vi "mmWave TX driver (FPGA).vi"() -> ()   [LabVIEW 2019]
uses:
  SubVIs/Tone Generator/Channel Control.ctl
  SubVIs/Sync/Sync Control.ctl
  SubVIs/Sync/Sync Measurements.ctl
  <instrlib>/_niInstr/DSP/v1/Shared/Public/IQ Impairments.ctl
  <instrlib>/_niInstr/DSP/v1/Shared/Public/Filter Coefficients.ctl
  Host/SubVIs/Low-level/TypeDefs/Gain Setting.ctl
  <instrlib>/niMmWave/ni3620/Config/v1/FPGA/Public/Typedefs/TX1 RX1 Port.ctl
  SubVIs/Utility/FPGA driver trigger destination.ctl
  SubVIs/Utility/FPGA driver trigger source.ctl
  SubVIs/DRAM burst sequencer/DRAM mode.ctl
  SubVIs/DRAM burst sequencer/SegementSequencer_class/FPGA sequencer states.ctl
  SubVIs/DRAM burst sequencer/Burst memo.ctl
  SubVIs/DRAM burst sequencer/DRAM resources.ctl
  <instrlib>/_niInstr/Memory/v1/FPGA/DRAM U512/niInstr Memory DRAM U512 v1 FPGA.lvclass
  <instrlib>/_niInstr/Memory/v1/FPGA/BRAM U512/niInstr Memory BRAM U512 v1 FPGA.lvclass
  <vilib>/Platform/TimedLoop/XDataNode/timing_clust.ctl
  <vilib>/Platform/TimedLoop/XDataNode/nitl_modes.ctl
  <vilib>/Platform/TimedLoop/XDataNode/wakeup.ctl
  <instrlib>/_niInstr/DSP/v1/Shared/Public/IQ Data.ctl
  <instrlib>/_niInstr/Memory/v1/FPGA/DRAM U512/Public/Create.vi
  <instrlib>/_niInstr/Memory/v1/FPGA/BRAM U512/Public/Create.vi
  <vilib>/rvi/Emulation/niFpgaSctlEmulationGetInTimedLoop.vi
  <vilib>/rvi/Emulation/niFpgaEmulationReportErrorSimple.vi
  <vilib>/rvi/Emulation/niFpgaGetClockAttributes.vi
  <vilib>/rvi/Emulation/niFpgaCriticalErrorInLSC.vi
  <vilib>/rvi/Emulation/niFpgaProcessEmulError.vi
  <vilib>/rvi/eio/common/nirviEmuTemplateMethod_errors.vi
  SubVIs/Misc/Globals.vi
  <vilib>/rvi/DataTransferAndStorage/Container/Common/niFpgaContainerGetUniqueNameForEmu.vi
  <vilib>/rvi/DataTransferAndStorage/Container/Common/niFpgaContainerSetEmuInfo.vi
  <vilib>/rvi/eio/common/nirviEmuReportErrorAndStop.vi
  <vilib>/rvi/Emulation/niFpgaEmulationIsFPGAContextNoSignature.vi
  <vilib>/rvi/errors/niFpgaSetErrorForExecOnDevCompSimple.vi
  <vilib>/rvi/FIFO/Fifo_Resource/nirvififoEmulationSetSize.vi
  <vilib>/rvi/FIFO/Fifo_Resource/nirviFifoEmulationQueueMgr.vi
  <instcachedir>/0/nirviFifoEmulationQueueMgr_E5CAEC123FF24DC58D834DCA3CDAA9B5.lvgen/nirviFifoEmulationQueueMgr_E5CAEC123FF24DC58D834DCA3CDAA9B5_008.vi
  <vilib>/Utility/error.llb/Clear Errors.vi
  <vilib>/rvi/FIFO/Fifo_Resource/nirvififoEmulationCreateLock.vi
  <vilib>/rvi/FIFO/Fifo_Resource/nirvififoEmulationObtainLock.vi
  <vilib>/rvi/FIFO/Fifo_Resource/nirvififoEmulationReleaseLock.vi
  <vilib>/rvi/occurrence/nirviWaitOnOccurrenceBase.vi
  <vilib>/rvi/errors/nirviReportUnexpectedCaseInternalError.vi
  <vilib>/rvi/errors/nirviReportUnexpectedCaseInternalError (U32).vi
  <vilib>/rvi/FIFO/Fifo_Resource/nirvififoEmulationDetermineInputValidOut.vi
  <vilib>/rvi/DataTransferAndStorage/Container/Common/niFpgaContainerExecOnDevCompGetState.vi
  <instcachedir>/0/nirviFifoEmulationQueueMgr_E5CAEC123FF24DC58D834DCA3CDAA9B5.lvgen/nirviFifoEmulationQueueMgr_E5CAEC123FF24DC58D834DCA3CDAA9B5_011.vi
  <vilib>/rvi/interface/RandomDataEmulation/niFpgaRandomDataHandleErrors.vi
  <instrlib>/_niInstr/Basic Elements/v1/FPGA/Private/Count Up U64.vi
  <vilib>/Platform/TimedLoop/XDataNode/XDataNode.xnode
  <vilib>/eio/EIONode/EIONode.xnode
  <vilib>/rvi/LocalResourceManager/LocalResourceManager.xnode
  <vilib>/rvi/DataTransferAndStorage/Container/XNode/niFpgaContainer.xnode
  <vilib>/rvi/FIFO/Fifo_Resource/nirvififoEmulationRead.vi
  <vilib>/rvi/FIFO/Fifo_Resource/nirvififoEmulationWrite.vi
  <vilib>/eio/EIOMethodNode/EIOMethodNode.xnode
  <vilib>/rvi/FIFO/Fifo_Resource/niFpgaFifoEmulationRefIn.vi
  SubVIs/DRAM burst sequencer/SegementSequencer_class/SegmentSequencer.lvclass
  <vilib>/Platform/TimedLoop/XDataNode/XDNodeRunTimeDep.lvlib
  <instrlib>/_niInstr/Basic Elements/v1/FPGA/niInstr Basic Elements v1 FPGA.lvlib
  <instrlib>/_niInstr/Data Formatting/v1/FPGA/niInstr Data Formatting v1 FPGA.lvlib
  <vilib>/rvi/Memory/Memory_Emulation/nirvimemoryFastEmulation.vi
  <vilib>/rvi/Memory/Memory_Emulation/nirvimemoryEmulation.vi
  <instrlib>/_niInstr/Basic Elements/v1/FPGA/Private/Count Up U16.vi
  <instrlib>/_niInstr/DSP/v1/Shared/niInstr DSP v1 Shared.lvlib
  <instrlib>/niMmWave/ni3620/Config/v1/FPGA/niMmWave Config v1 FPGA.lvlib
  <vilib>/rvi/interface/RandomDataEmulation/nirviRandomDataFpgaMultiElementTemplate.vi
  SubVIs/Utility/FPGA Utility.lvlib
  <instrlib>/_niInstr/Memory/v1/FPGA/DRAM/niInstr Memory DRAM v1 FPGA.lvclass
  SubVIs/DRAM burst sequencer/TX burst sequencer.lvlib
  <instrlib>/_niInstr/Memory/v1/FPGA/BRAM/niInstr Memory BRAM v1 FPGA.lvclass
  <instrlib>/_niInstr/Data Formatting/v1/FPGA/Private/Convert/U32 array to Boolean Array.vi
  <instrlib>/_niInstr/Data Formatting/v1/FPGA/Private/Convert/Boolean Array to U32 Array.vi
panel:
  in  "gen.enable":bool
  out "bram.last written addr":u32
  out "bram.debug ctr":T1
  in  "burst memo":T2
  out "flush":bool
  out "gen.total samples":u64
  out "gen.pending to read":u32
  in  "seq.start":bool
  in  "seq.rst":bool
  out "seq.state":T3
  out "seq.step ctr":u32
  out "seq.repeat ctr":u64
  out "seq.loaded steps":u32
  out "seq.req ctr":i64
  in  "seq.continous":bool
  in  "seq.add step":bool
  in  "seq.new step":T4
  in  "memo.reset":bool
  in  "memo.ctr rst":bool
  out "dram.last written addr":u32
  out "dram.debug ctr":T1
  in  "memo mode":T5
  in  "iq.load":bool
  in  "iq.load addr":u32
  out "aurora.data":u16
  out "aurora.trig count":u16
  in  "trig.pxi dst":i32
  out "pxi.trig count":u16
  in  "trig.pxi src":i32
  in  "trig.source":T6
  in  "trig.export dur":u32=25
  in  "gen.burst/cont":bool
  out "aurora.tx val":u16
  in  "trig.export":T7
  in  "trig.delay":u16
  in  "sync.master reset listen":bool
  in  "sync.counter reset enable":bool
  in  "20 kHz tclk parameters":T8
  out "sysref value":u8
  out "tclk value":u16
  in  "gain ranging.enable port config":bool
  in  "gain ranging.enable coarse gain ranging":bool
  in  "gain ranging.enable fine gain ranging":bool
  in  "gain ranging.coarse gain values":fxp<+/-,16,12>[](array[numeric])=[0.0, 0.0, 0.0, 0.0]
  out "port 5.debug info":T9
  out "port 5.rx fifo overflow":bool
  in  "port 5.rx fifo overflow clear":bool
  out "port 4.rx fifo overflow":bool
  in  "port 4.rx fifo overflow clear":bool
  out "port 4.debug info":T9
  out "aurora.fifo 1 overflow":bool
  in  "aurora.reset trigger":bool
  out "aurora.fifo 0 overflow":bool
  in  "aurora.fifo overflow clear":bool
  in  "aurora.write":bool
  out "clocks valid":bool[](array[boolean])
  in  "table info":T10
  in  "gain ranging.manual setting":T13
  in  "gain ranging.setting list step":T14
  in  "gain ranging.enable":bool
  in  "gain ranging.dwell time (cycles)":u32=4800
  in  "txjesd.control":T15
  out "txjesd.status":T16
  in  "filter.enable":bool
  in  "filter.coefficients":T17
  in  "cal.correction":T19={"sample delay"={"I delay"=0.0, "Q delay"=0.0}, "fractional delay"={"enable"=FALSE, "coef write"=FALSE, "coef data"=0.0}, "impairments"={"inline gain I"=0.9999923706054688, "inline gain Q"=0.9999923706054688, "cross gain I"=0.0, "cross gain Q"=0.0, "pre-gain offset I"=0.0, "pre-gain offset Q"=0.0, "post-gain offset I"=0.0, "post-gain offset Q"=0.0}, "iq inversion"={"invert I"=FALSE, "invert Q"=FALSE}}
  out "sync.measurements":T20
  in  "sync.parameters":T22
  in  "sync.use synced trigger":bool
  in  "sync.trigger":bool
  in  "gen.read":bool
  in  "cal.generation":T23={"generation select"=enum."Pass Through", "tone parameters"={"frequency"=0.125, "gain"=0.5}, "pulse parameters"={"frequency"=16, "gain"=0.5, "width"=16}}
  in  "gen.load":bool
  in  "gen.triggered read":bool
  in  "gen.length":u16=15
  in  "gen.write enable":bool
  in  "tone.routing":cluster{"I":T24, "Q":T24}
  in  "tone.parameters":T25(array[cluster])=[{"frequency"=0.032551999999999026, "gain"=0.8000030517578125, "phase"=0.0, "offset"={"offset I"=0.0, "offset Q"=0.0}}, {"frequency"=0.032551999999999026, "gain"=0.0, "phase"=0.0, "offset"={"offset I"=0.0, "offset Q"=0.0}}] {"offset"."offset Q" format="%#.18g"; "offset"."offset I" format="%#.18g"}
  in  "waveform type":enum16{"Tone", "Waveform Generation"}(ring)
  # "TX Generation"
  # "TX BURST GEN"
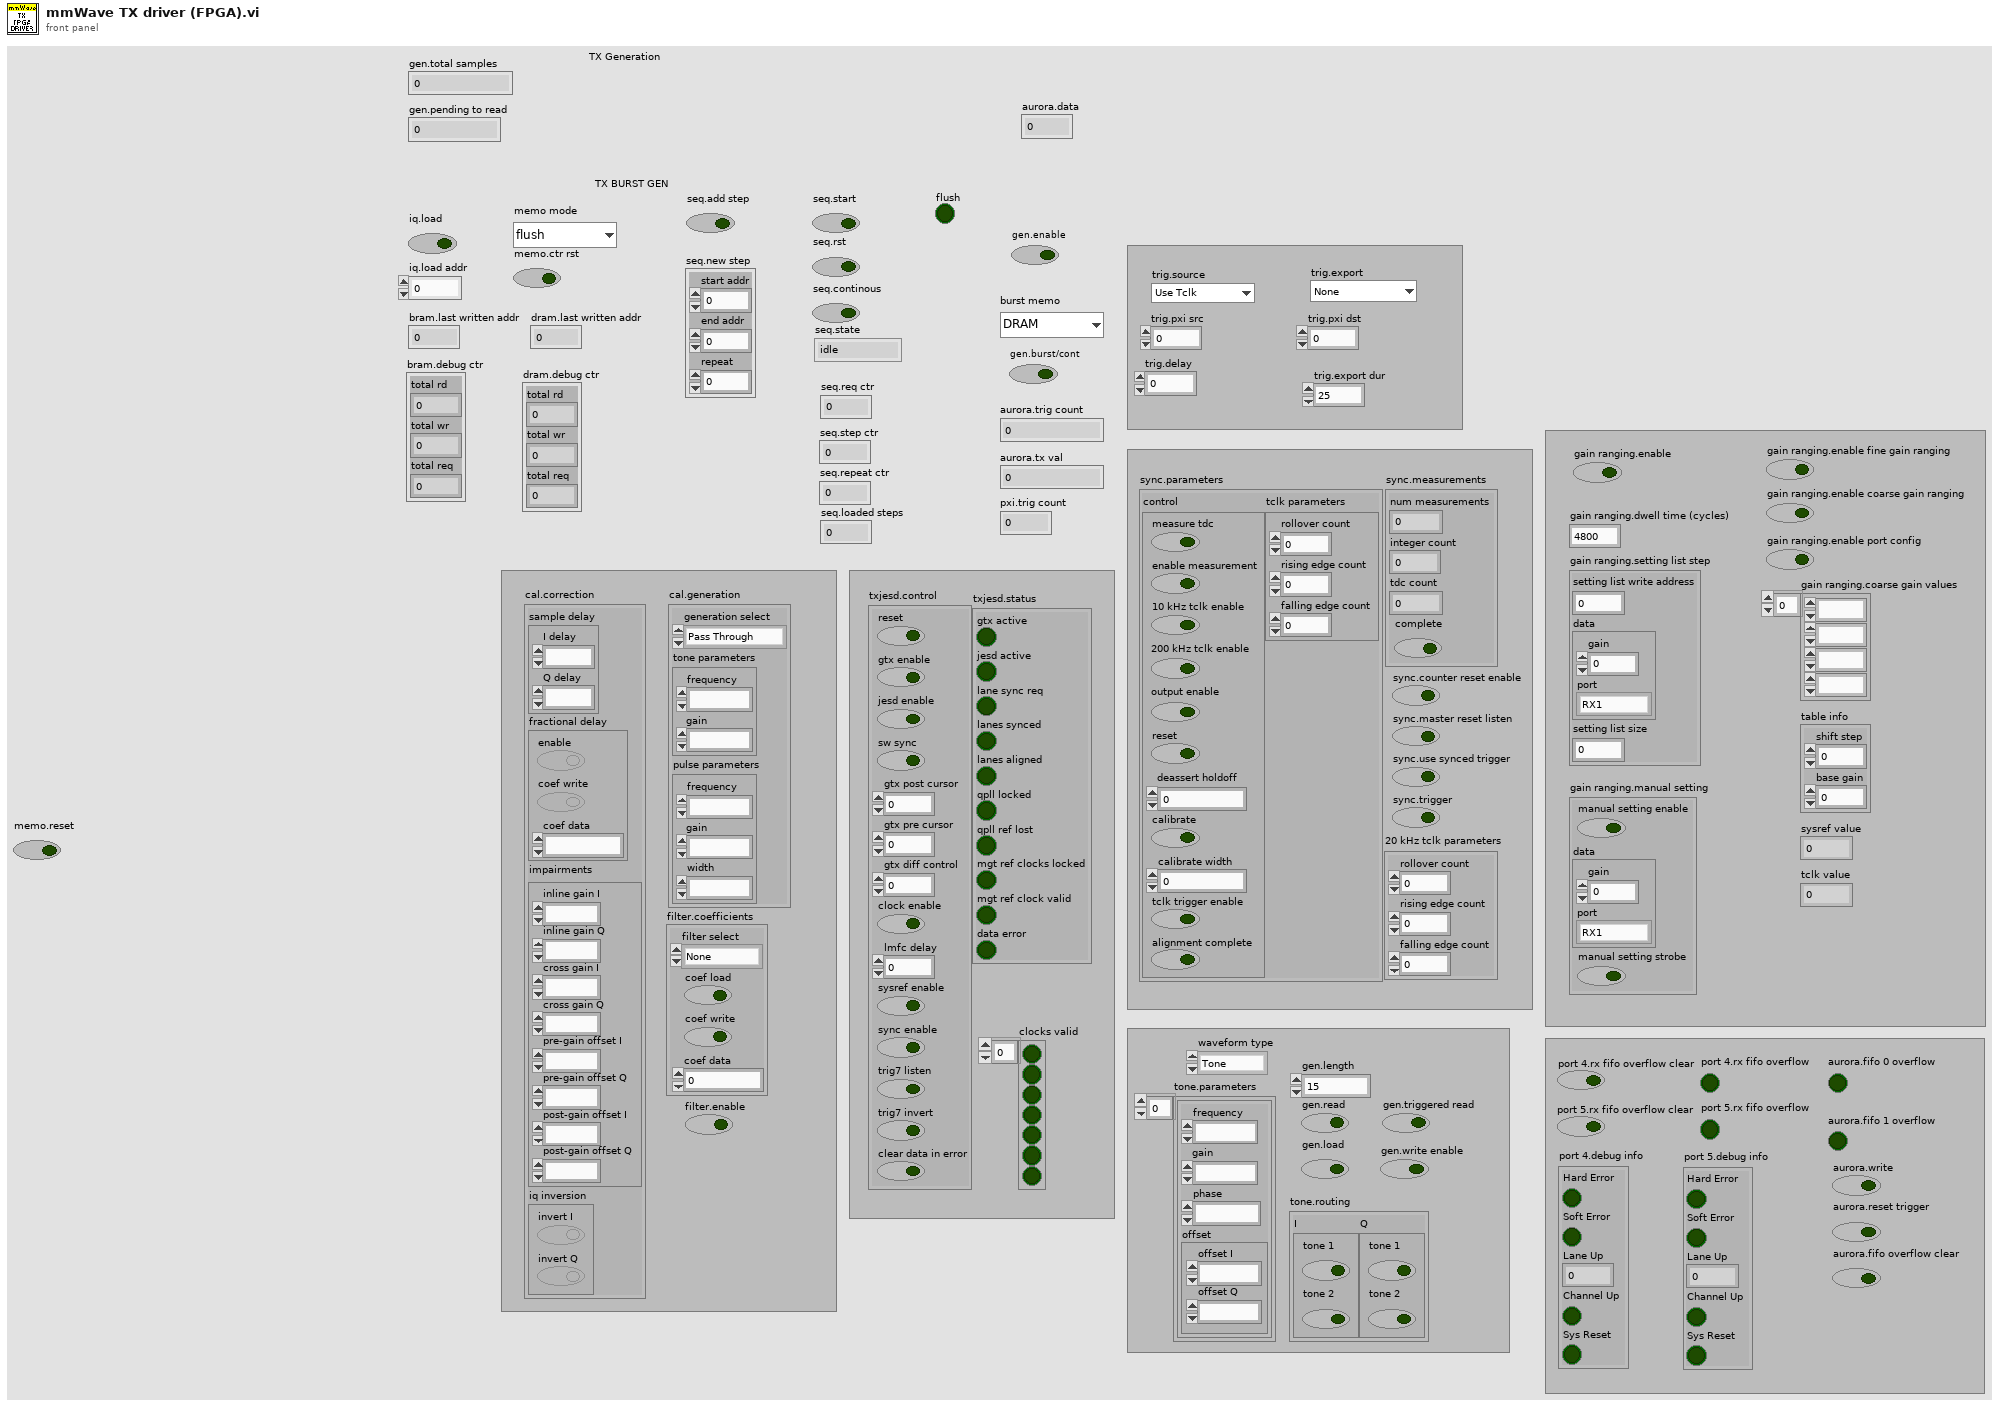
[diagram p1: front panel]
types:
  T1 = cluster{"total rd":u32, "total wr":u32, "total req":u32}
  T2 = typedef "TX burst sequencer.lvlib/Burst memo.ctl" = enum16{"DRAM", "BRAM"}
  T3 = typedef "FPGA sequencer states.ctl" = enum16{"idle", "read step", "execute step"}
  T4 = cluster{"start addr":u32, "end addr":u32, "repeat":u64}
  T5 = typedef "TX burst sequencer.lvlib/DRAM mode.ctl" = enum16{"flush", "reset", "write", "read"}
  T6 = typedef "FPGA Utility.lvlib/FPGA driver trigger source.ctl" = enum16{"Use Tclk", "PXI_Trig", "Aurora RX trig"}
  T7 = typedef "FPGA Utility.lvlib/FPGA driver trigger destination.ctl" = enum16{"None", "Source trig", "Synced trig", "Delayed sync"}
  T8 = cluster{"rollover count":u16, "rising edge count":u16, "falling edge count":u16}
  T9 = cluster{"Hard Error":bool, "Soft Error":bool, "Lane Up":fxp<+,4,4>, "Channel Up":bool, "Sys Reset":bool}
  T10 = cluster{"shift step":i16, "base gain":fxp<+/-,16,12>}
  T11 = typedef "gain setting.ctl" = cluster{"gain":fxp<+/-,16,12>, "port":T12}
  T12 = typedef "TX1 RX1 Port.ctl" = enum8{"RX1", "TX1/RX2"}
  T13 = cluster{"manual setting enable":bool, "data":T11, "manual setting strobe":bool}
  T14 = cluster{"setting list write address":u32, "data":T11, "setting list size":u16}
  T15 = cluster{"reset":bool, "gtx enable":bool, "jesd enable":bool, "sw sync":bool, "gtx post cursor":fxp<+,5,5>, "gtx pre cursor":fxp<+,5,5>, "gtx diff control":fxp<+,4,4>, "clock enable":bool, "lmfc delay":fxp<+,5,5>, "sysref enable":bool, "sync enable":bool, "trig7 listen":bool, "trig7 invert":bool, "clear data in error":bool}
  T16 = cluster{"gtx active":bool, "jesd active":bool, "lane sync req":bool, "lanes synced":bool, "lanes aligned":bool, "qpll locked":bool, "qpll ref lost":bool, "mgt ref clocks locked":bool, "mgt ref clock valid":bool, "data error":bool}
  T17 = typedef "niInstr DSP v1 Shared.lvlib/Filter Coefficients.ctl" = cluster{"filter select":enum8{"None", "I Inline", "I Cross", "Q Cross", "Q Inline"}, "coef load":bool, "coef write":bool, "coef data":fxp<+/-,18,1>}
  T18 = typedef "niInstr DSP v1 Shared.lvlib/IQ Impairments.ctl" = cluster{"inline gain I":fxp<+/-,18,1>, "inline gain Q":fxp<+/-,18,1>, "cross gain I":fxp<+/-,18,1>, "cross gain Q":fxp<+/-,18,1>, "pre-gain offset I":fxp<+/-,18,1>, "pre-gain offset Q":fxp<+/-,18,1>, "post-gain offset I":fxp<+/-,18,1>, "post-gain offset Q":fxp<+/-,18,1>}
  T19 = cluster{"sample delay":cluster{"I delay":fxp<+,13,13>, "Q delay":fxp<+,13,13>}, "fractional delay":cluster{"enable":bool, "coef write":bool, "coef data":fxp<+/-,18,1>}, "impairments":T18, "iq inversion":cluster{"invert I":bool, "invert Q":bool}}
  T20 = typedef "Sync Measurements.ctl" = cluster{"num measurements":u16, "integer count":u16, "tdc count":u16, "complete":bool}
  T21 = typedef "Sync Control.ctl" = cluster{"measure tdc":bool, "enable measurement":bool, "10 kHz tclk enable":bool, "200 kHz tclk enable":bool, "output enable":bool, "reset":bool, "deassert holdoff":u8, "calibrate":bool, "calibrate width":u8, "tclk trigger enable":bool, "alignment complete":bool}
  T22 = cluster{"control":T21, "tclk parameters":cluster{"rollover count":u16, "rising edge count":u16, "falling edge count":u16}}
  T23 = cluster{"generation select":enum16{"Pass Through", "Tone", "Pulse", "Disable"}, "tone parameters":cluster{"frequency":fxp<+/-,48,0>, "gain":fxp<+/-,18,1>}, "pulse parameters":cluster{"frequency":u32, "gain":fxp<+/-,18,1>, "width":u8}}
  T24 = typedef "Channel Control.ctl" = cluster{"tone 1":bool, "tone 2":bool}
  T25 = cluster{"frequency":fxp<+/-,48,0>, "gain":fxp<+/-,18,1>, "phase":fxp<+/-,21,0>, "offset":cluster{"offset I":fxp<+/-,18,1>, "offset Q":fxp<+/-,18,1>}}[]
  T26 = typedef "TX burst sequencer.lvlib/DRAM resources.ctl" = cluster{"DRAM read data FIFO":refnum<k21>, "DRAM write data FIFO":refnum<k21>, "DRAM request FIFO":refnum<k21>, "DRAM U512 memo":refnum<class "niInstr Memory DRAM U512 v1 FPGA.lvclass">, "DMA data loader":refnum<k21>, "BRAM read data FIFO":refnum<k21>, "BRAM write data FIFO":refnum<k21>, "BRAM request FIFO":refnum<k21>, "BRAM U512 memo":refnum<class "niInstr Memory BRAM U512 v1 FPGA.lvclass">}
  T27 = cluster{"s_axis_tvalid":refnum<k21>, "s_axis_tdata_0":refnum<k21>, "s_axis_tdata_1":refnum<k21>, "s_axis_tdata_2":refnum<k21>, "s_axis_tdata_3":refnum<k21>, "s_axis_tready":refnum<k21>}
  T28 = cluster{"m_axis_tvalid":refnum<k21>, "m_axis_tdata_0":refnum<k21>, "m_axis_tdata_1":refnum<k21>, "m_axis_tdata_2":refnum<k21>, "m_axis_tdata_3":refnum<k21>}
  T29 = typedef "XDNodeRunTimeDep.lvlib/timing_clust.ctl" = cluster{"Expected End [f-1]":u64, "Actual End [f-1]":u64, "Finished Late? [f-1]":bool, "Expected End [i-1]":u64, "Actual End [i-1]":u64, "Finished Late? [i-1]":bool, "Expected Start [i]":u64, "Actual Start [i]":u64, "Expected Start [f]":u64, "Actual Start [f]":u64, "Source Name":string, "Structure Name":string, "Period":i64, "Deadline":i64, "Offset":i64, "Start":i64, "Priority":i32, "Timeout":i32, "Mode":T30, "Wakeup Reason":T31, "Error":errorcluster, "Source Type":string, "Secondary Source Type":string, "Global End Time":u64, "Global Start Time":u64, "Frame Duration":u64, "Iteration Duration":u64, "Assigned CPU":i32, "I/O Scan Engine Mode":u32}
  T30 = typedef "XDNodeRunTimeDep.lvlib/nitl_modes.ctl" = enum32{"No Change", "Process missed periods, maintain original phase", "Discard missed periods, maintain original phase", "Process missed periods, ignore original phase", "Discard missed periods, ignore original phase"}
  T31 = typedef "XDNodeRunTimeDep.lvlib/wakeup.ctl" = enum32{"Normal", "Aborted", "Asynchronous wakeup", "Timing source error", "Timed loop error", "Timeout"}
  T32 = typedef "Sync Resources.ctl" = cluster{"tdc assert":refnum<k21>, "tdc deassert":refnum<k21>, "tdc count":refnum<k21>, "control":refnum<k21>, "integer count":refnum<k21>}
  T33 = typedef "AXI4-Stream Reader FXP64x4 Resources.ctl" = cluster{"AXI4-Stream Reader Resources":cluster{"Use TREADY":bool, "Use TLAST":bool, "TLAST":refnum<k21>, "TREADY":refnum<k21>, "TVALID":refnum<k21>, "Use TKEEP":bool, "Use TSTRB":bool, "Use TUSER":bool}, "TDATA Resources":cluster{"TDATA_0":refnum<k21>, "TDATA_1":refnum<k21>, "TDATA_2":refnum<k21>, "TDATA_3":refnum<k21>}, "TKEEP":refnum<k21>, "TSTRB":refnum<k21>}
  T34 = typedef "AXI4-Stream Writer FXP64x4 Resources.ctl" = cluster{"Writer Resources":cluster{"Use TREADY":bool, "Use TLAST":bool, "TLAST":refnum<k21>, "TREADY":refnum<k21>, "TVALID":refnum<k21>, "Use TSTRB":bool, "Use TKEEP":bool, "Use TUSER":bool}, "TDATA Resources":cluster{"TDATA_0":refnum<k21>, "TDATA_1":refnum<k21>, "TDATA_2":refnum<k21>, "TDATA_3":refnum<k21>}, "TKEEP":refnum<k21>, "TSTRB":refnum<k21>}
  T35 = typedef "niInstr DSP v1 Shared.lvlib/IQ Data.ctl" = cluster{"I":fxp<+/-,18,1>, "Q":fxp<+/-,18,1>, "overflow":bool}
  T36 = cluster{"disable TClk measure":bool, "output enable":bool, "output value":bool}
  T37 = cluster{"Hard Error":refnum<k21>, "Soft Error":refnum<k21>, "Lane Up":refnum<k21>, "Channel Up":refnum<k21>, "Sys Reset":refnum<k21>}
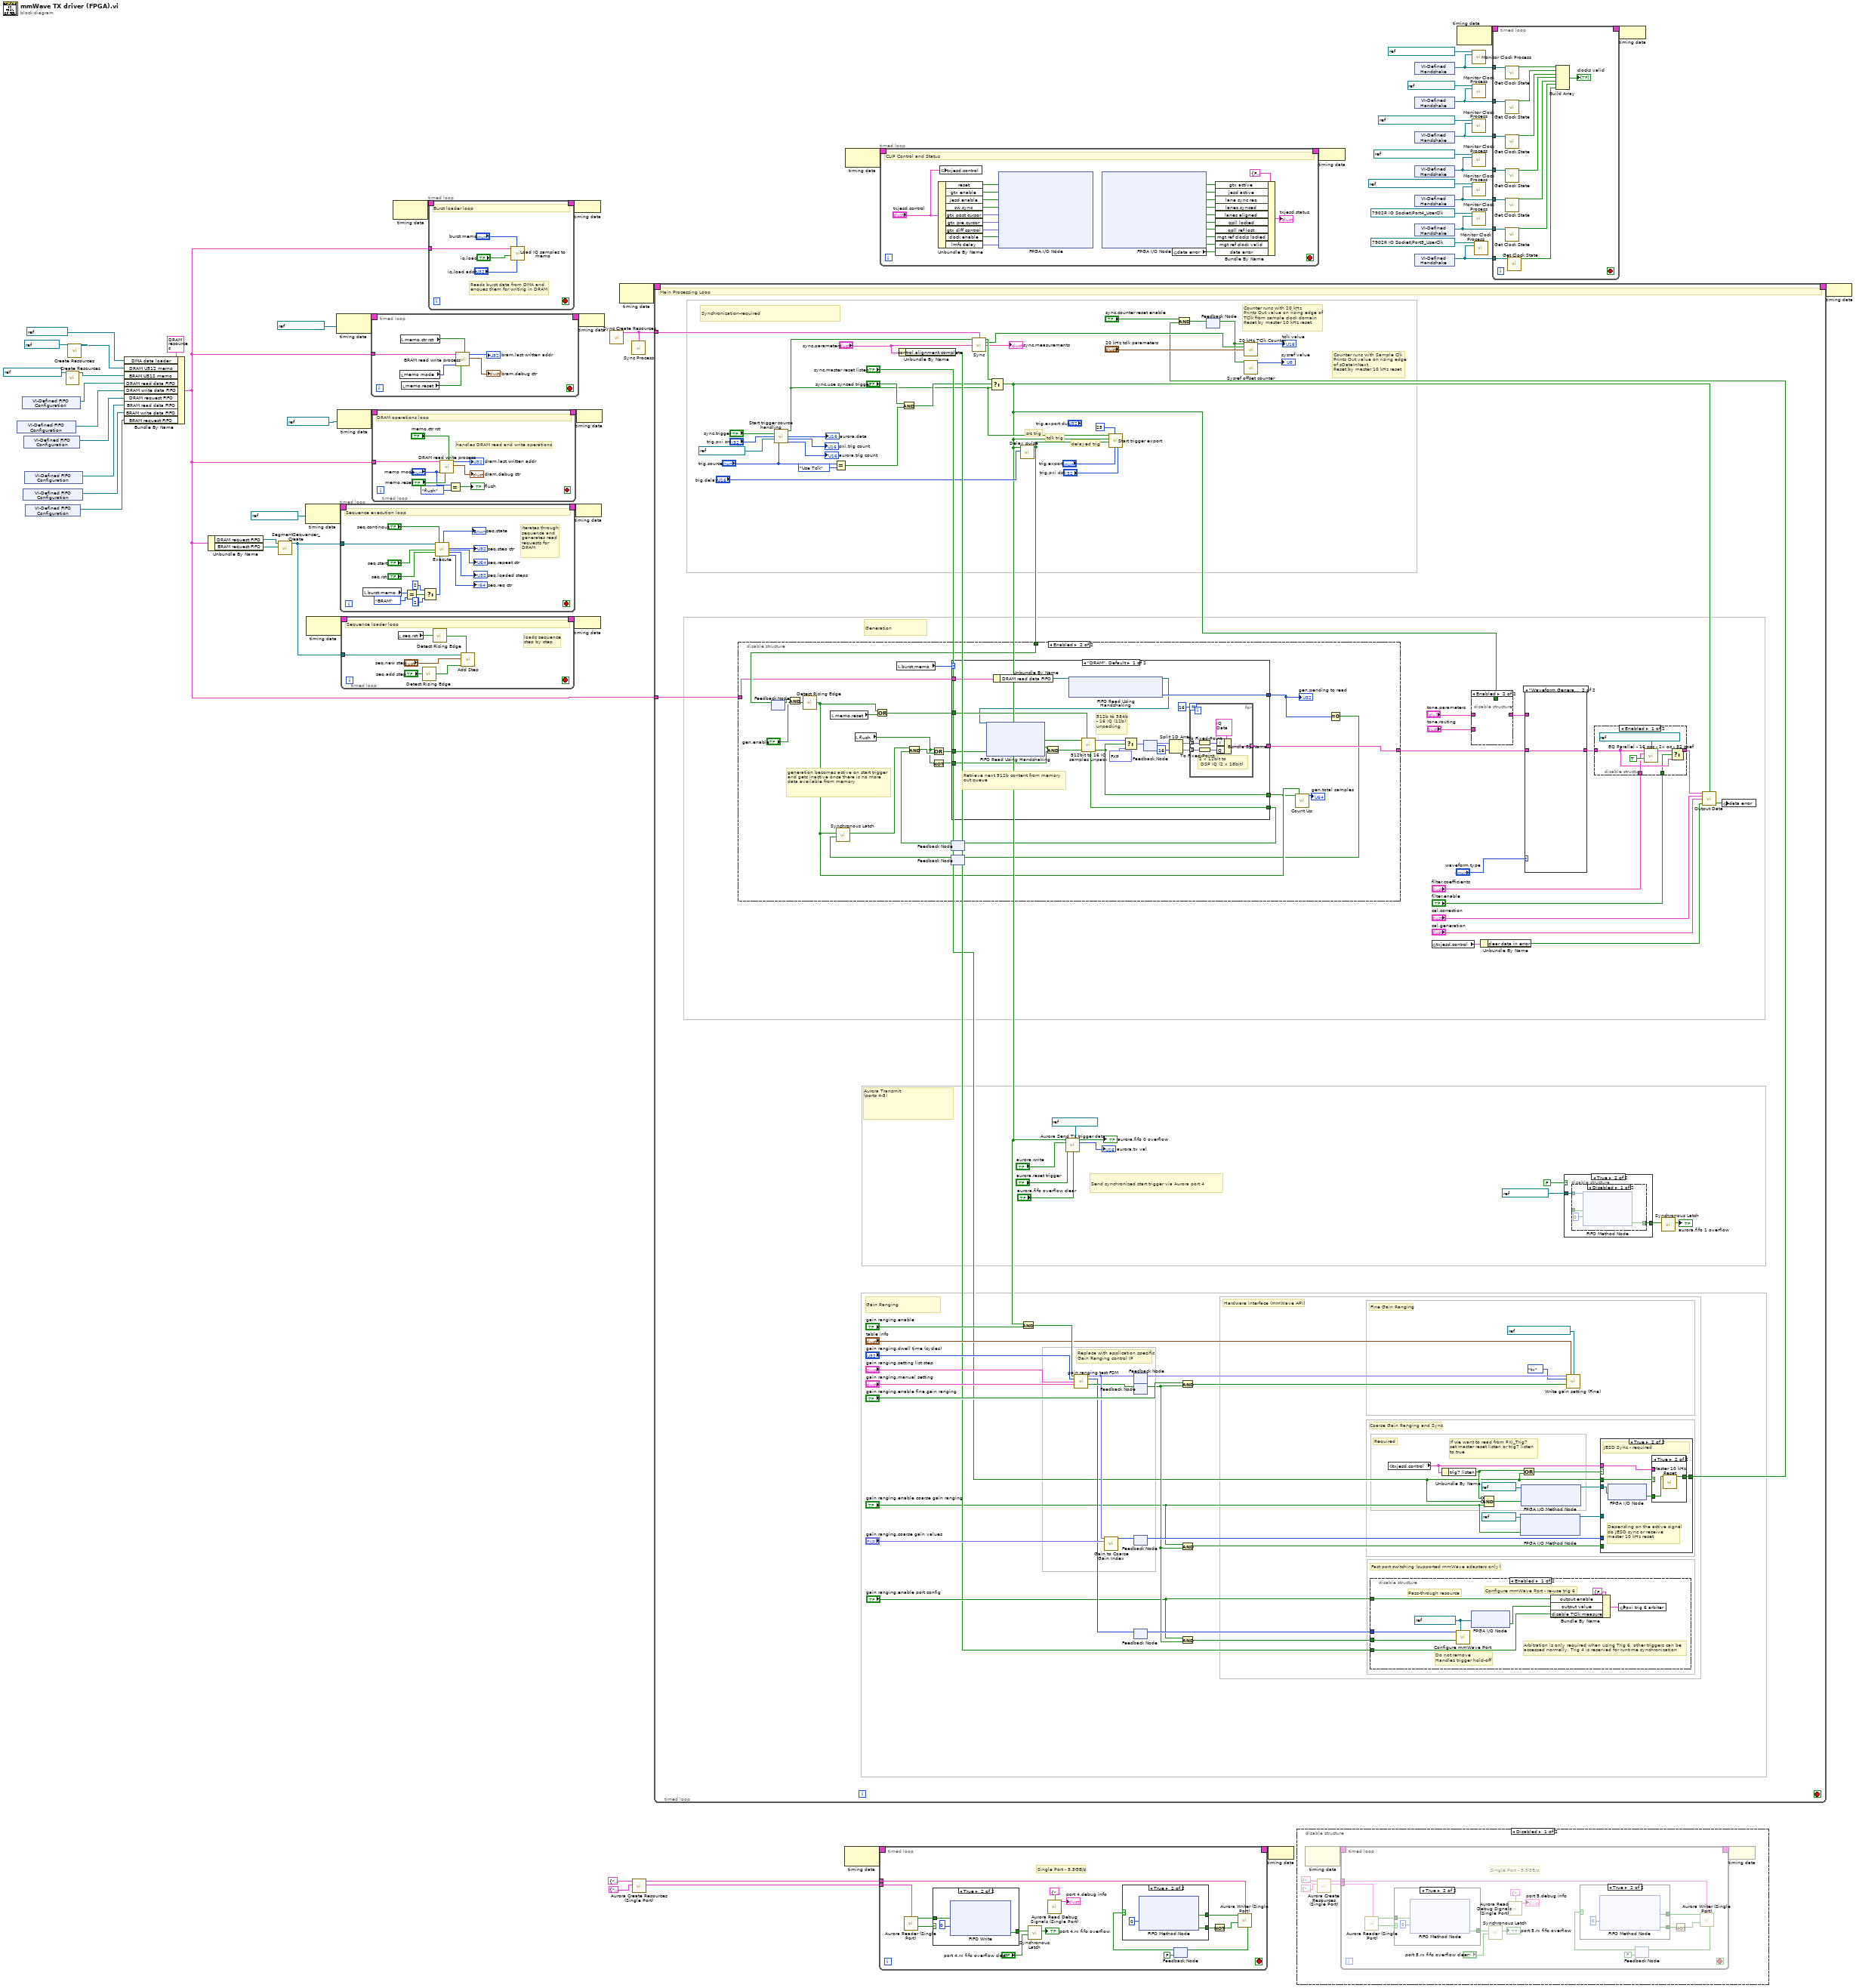
[diagram p0: block diagram]
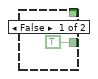
[diagram p2: hidden frame]
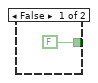
[diagram p3: hidden frame]
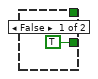
[diagram p5: hidden frame]
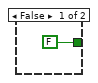
[diagram p6: hidden frame]
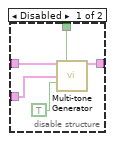
[diagram p7: hidden frame]
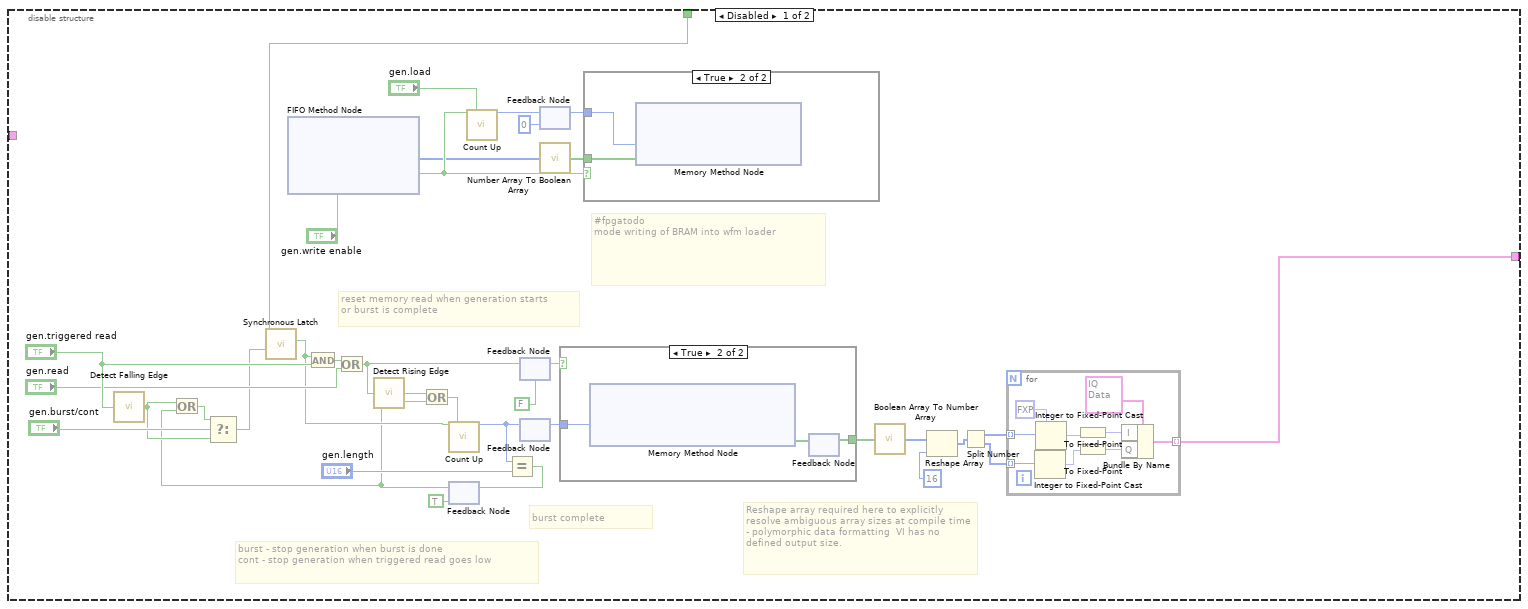
[diagram p10: hidden frame]
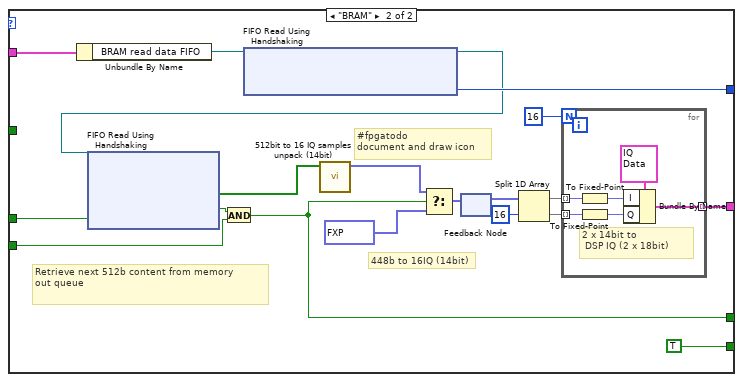
[diagram p13: hidden frame]
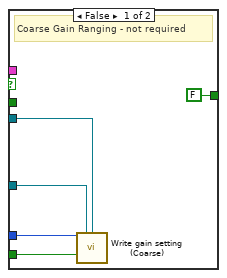
[diagram p14: hidden frame]
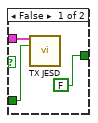
[diagram p15: hidden frame]
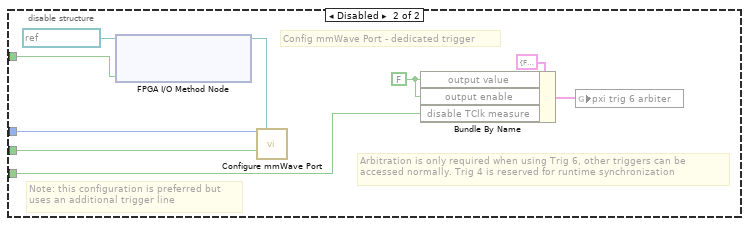
[diagram p16: hidden frame]
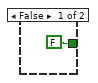
[diagram p17: hidden frame]
diagram:
  n1 = xnode "VI-Defined FIFO Configuration"() -> ("FIFO Out"=w26:refnum<k21>)
  n2 = xnode "VI-Defined FIFO Configuration"() -> ("FIFO Out"=w27:refnum<k21>)
  n3 = xnode "VI-Defined FIFO Configuration"() -> ("FIFO Out"=w10:refnum<k21>)
  n4 = xnode "VI-Defined FIFO Configuration"() -> ("FIFO Out"=w25:refnum<k21>)
  n5 = xnode "VI-Defined FIFO Configuration"() -> ("FIFO Out"=w11:refnum<k21>)
  n6 = xnode "VI-Defined FIFO Configuration"() -> ("FIFO Out"=w9:refnum<k21>)
  n7 = call-poly <instrlib>:"Create Resources.vi"("memory in"=refnum<k21> "generation memory") -> ("memory out"=w1:refnum<class "niInstr Memory BRAM U512 v1 FPGA.lvclass">)  [unwired: 14 in]
  n8 = call-poly <instrlib>:"Create Resources.vi"("memory in"=refnum<k21> "TX memo") -> ("memory out"=w24:refnum<class "niInstr Memory DRAM U512 v1 FPGA.lvclass">)  [unwired: 14 in]
  n9 = Bundle By Name(cluster=T26 {"DRAM read data FIFO"="", "DRAM write data FIFO"="", "DRAM request FIFO"="", "DRAM U512 memo"=refnum, "DMA data loader"="custom data", "BRAM read data FIFO"="", "BRAM write data FIFO"="", "BRAM request FIFO"="", "BRAM U512 memo"=refnum} ("DRAM resources"), "DMA data loader"=refnum<k21> "custom data" ("FIFO In"), "DRAM U512 memo"=w24, "BRAM U512 memo"=w1, "DRAM read data FIFO"=w27, "DRAM write data FIFO"=w26, "DRAM request FIFO"=w25, "BRAM read data FIFO"=w11, "BRAM write data FIFO"=w10, "BRAM request FIFO"=w9) -> (w3:T26)
  n10 = Unbundle By Name(w3) -> ("DRAM request FIFO"=w5:refnum<k21>, "BRAM request FIFO"=w4:refnum<k21>)
  n11 = call "SegmentSequencer_Create.vi"("req fifo 2"=w4, "req fifo 1"=w5) -> ("New SegmentSequencer"=w12:refnum<class "SegmentSequencer.lvclass">)  [unwired: 9 in]
  n12 = node-c288(refnum<k21> "200 MHz Clock" ("Source Name")) -> (w15:T29)
  n13 = node-c288() -> (w17:T29)  [unwired: 1 in]
  n14 = node-c288(refnum<k21> "200 MHz Clock" ("Source Name")) -> (w8:T29)
  n15 = node-c288(refnum<k21> "DRAM Clock" ("Source Name")) -> (w20:T29)
  n16 = timed-loop {
    timing: w15 -> [_]
    timing-out: [_] -> w14
    tunnel: w12 -> [w65]
    stop <- _ stop-if-true
    (unwired) i16 2 ("req fifo")
    # "iterates through\nsequence and\ngenerates read\nrequests for\nDRAM"
    # "Sequence execution loop"
    n17 = local read "burst memo"() -> (w62:T2)
    n18 = Equal?(x=w62, y=Burst_memo."BRAM") -> (x = y?=w60:bool)
    n19 = Select(t=i16 2 ("req fifo"), s=w60, f=i16 1 ("req fifo")) -> (s? t:f=w57:i16)
    n20 = call-dynamic "Execute.vi"("SegmentSequencer in"=w65, "start"="seq.start", "reset"="seq.rst", "continuous?"="seq.continous", "req fifo"=w57) -> ("state"=→"seq.state":T3, "step counter"=→"seq.step ctr":u32, "repeat counter"=→"seq.repeat ctr":u64, "Loaded steps"=→"seq.loaded steps":u32, "generated requests"=→"seq.req ctr":i64)  [unwired: 9 in, 1 out]
  }
  n21 = timed-loop {
    timing: w17 -> [_]
    timing-out: [_] -> w16
    tunnel: w12 -> [w79]
    stop <- _ stop-if-true
    # "loads sequence\nstep by step"
    # "Sequence loader loop"
    n22 = local read "seq.rst"() -> (w75:bool)
    n23 = call <instrlib>:"Detect Rising Edge.vi"("signal"="seq.add step") -> ("edge detected"=w78:bool)  [unwired: 14 in]
    n24 = call <instrlib>:"Detect Rising Edge.vi"("signal"=w75) -> ("edge detected"=w74:bool)  [unwired: 14 in]
    n25 = call-dynamic "Add Step.vi"("reset load"=w74, "input valid"=w78, "Data"="seq.new step", "SegmentSequencer in"=w79) -> ()  [unwired: 7 in, 1 out]
  }
  n26 = timed-loop {
    timing: w8 -> [_]
    timing-out: [_] -> w7
    tunnel: w3 -> [w87]
    stop <- _ stop-if-true
    n27 = local read "memo mode"() -> (w86:T5)
    n28 = local read "memo.ctr rst"() -> (w84:bool)
    n29 = local read "memo.reset"() -> (w85:bool)
    n30 = call "BRAM read write process.vi"("debug ctr reset"=w84, "dram.reset"=w85, "dram mode"=w86, "DRAM resources"=w87) -> ("BRAM debug ctr"=→"bram.debug ctr":T1, "last written addr"=→"bram.last written addr":u32)  [unwired: 6 in]
  }
  n31 = timed-loop {
    timing: w20 -> [_]
    timing-out: [_] -> w19
    tunnel: w3 -> [w93]
    stop <- _ stop-if-true
    # "handles DRAM read and write operations"
    # "DRAM operations loop"
    n32 = call "DRAM read write process.vi"("debug ctr reset"="memo.ctr rst", "dram.reset"="memo.reset", "dram mode"="memo mode", "DRAM resources"=w93) -> ("DRAM debug ctr"=→"dram.debug ctr":T1, "last written addr"=→"dram.last written addr":u32)  [unwired: 6 in]
    n33 = Equal?(x="memo mode", y=DRAM_mode."flush") -> (x = y?=→"flush":bool)
  }
  n34 = node-c288() -> (w22:T29)  [unwired: 1 in]
  n35 = timed-loop {
    timing: w22 -> [_]
    timing-out: [_] -> w21
    tunnel: w3 -> [w101]
    stop <- _ stop-if-true
    # "Reads burst data from DMA and\nenques them for writing in DRAM"
    # "Burst loader loop"
    n36 = call "Load IQ samples to memo.vi"("wr.start addr"="iq.load addr", "burst memo"="burst memo", "wr.enable"="iq.load", "DRAM resources"=w101) -> ()  [unwired: 8 in]
  }
  n37 = node-c288(w21) -> ()
  n38 = node-c288(w16) -> ()
  n39 = node-c288(w14) -> ()
  n40 = node-c288(w19) -> ()
  n41 = node-c288(w7) -> ()
  n42 = call "Sync Create Resources.vi"() -> ("sync.resources"=w52:T32)  [unwired: 15 in]
  n43 = node-c288() -> (w54:T29)  [unwired: 1 in]
  n44 = call "Sync Process.vi"("sync.resources"=w52) -> ()  [unwired: 15 in]
  n45 = call "Aurora Create Resources (Single Port).vi"("RX CLIP Resources"=T28 {"m_axis_tvalid"="7902R IO Socket\\uPort4_m_axi_rx_tvalid", "m_axis_tdata_0"="7902R IO Socket\\uPort4_m_axi_rx_tdata_0", "m_axis_tdata_1"="7902R IO Socket\\uPort4_m_axi_rx_tdata_1", "m_axis_tdata_2"="7902R IO Socket\\uPort4_m_axi_rx_tdata_2", "m_axis_tdata_3"="7902R IO Socket\\uPort4_m_axi_rx_tdata_3"}, "TX CLIP Resources"=T27 {"s_axis_tvalid"="7902R IO Socket\\uPort4_s_axi_tx_tvalid", "s_axis_tdata_0"="7902R IO Socket\\uPort4_s_axi_tx_tdata_0", "s_axis_tdata_1"="7902R IO Socket\\uPort4_s_axi_tx_tdata_1", "s_axis_tdata_2"="7902R IO Socket\\uPort4_s_axi_tx_tdata_2", "s_axis_tdata_3"="7902R IO Socket\\uPort4_s_axi_tx_tdata_3", "s_axis_tready"="7902R IO Socket\\uPort4_s_axi_tx_tready"}) -> ("AXI4-Stream Reader FXP64x4"=w33:T33, "AXI4-Stream Writer FXP64x4"=w32:T34)  [unwired: 8 in]
  n46 = timed-loop {
    timing: w54 -> [_]
    timing-out: [_] -> w53
    tunnel: w52 -> [w151]
    tunnel: w3 -> [w116]
    stop <- _ stop-if-true
    # "delayed trig"
    # "tclk trig"
    # "src trig"
    # "Send synchronized start trigger via Aurora port 4"
    # "Counter runs with Sample Clk\nPrints Out value on rising edge\nof sDataInNext\nReset by master 10 kHz reset"
    # "If we want to read from PXI_Trig7\nset master reset listen or trig7 listen\nto true"
    # "Counter runs with 20 kHz\nPrints Out value on rising edge of \nTClk from sample clock domain\nReset by master 10 kHz reset"
    # "Replace with application specific Gain Ranging control IP"
    # "Fast port switching (supported mmWave adapters only)"
    # "Fine Gain Ranging"
    # "Gain Ranging"
    # "Synchronization-required"
    # "Aurora Transmit\n(ports 4-5)"
    # "Hardware interface (mmWave API)"
    # "Generation"
    # "Coarse Gain Ranging and Sync"
    # "Required"
    # "Required"
    # "Main Processing Loop"
    n47 = call "Start trigger source handling.vi"("sync.trigger"="sync.trigger", "trig.pxi trig src"="trig.pxi src", "Refnum in"=refnum<k21> "aurora rx fifo 0" ("FIFO In"), "trig.source"="trig.source") -> ("trigger"=w118:bool, "aurora.data"=→"aurora.data":u16, "pxi.trig count"=→"pxi.trig count":u16, "aurora.trig count"=→"aurora.trig count":u16)  [unwired: 8 in]
    n48 = Equal?(x="trig.source", y=FPGA_driver_trigger_source."Use Tclk") -> (x = y?=w120:bool)
    n49 = Unbundle By Name("sync.parameters") -> ("control.alignment complete"=w154:bool)
    n50 = And(x="sync.use synced trigger", y=w120) -> (x .and. y?=w119:bool)
    n51 = call "Sync.vi"("trigger"=w118, "sync.resources"=w151, "sync.parameters"="sync.parameters") -> ("synced trigger"=w192:bool, "tclk"=w153:bool, "sync measurements"=→"sync.measurements":T20)  [unwired: 10 in]
    n52 = Select(t=w192, s=w119, f=w118) -> (s? t:f=w107:bool)
    n53 = call "Delay pulse.vi"("delay"="trig.delay", "signal in"=w107) -> ("delayed rising edge"=w117:bool)  [unwired: 9 in]
    n54 = disable-structure shown="Enabled" {
      disable-tunnel: [w209 w270] -> w106
      disable-tunnel: w117 -> [w210 w274]
      disable-tunnel: w116 -> [_ w266]
      frame Disabled {
        # "#fpgatodo\nmode writing of BRAM into wfm loader"
        # "reset memory read when generation starts\nor burst is complete"
        # "burst complete"
        # "burst - stop generation when burst is done\ncont - stop generation when triggered read goes low"
        # "Reshape array required here to explicitly resolve ambiguous array sizes at compile time - polymorphic data formatting  VI has no defined output size."
        n55 = call <instrlib>:"Detect Falling Edge.vi"("signal"="gen.triggered read") -> ("edge detected"=w213:bool)  [unwired: 14 in]
        n56 = xnode ("FIFO Method Node")("Ready for Output"="gen.write enable") -> ("Element"=w227:u32[], "Output Valid"=w232:bool)  [unwired: 1 in, 1 out]
        n57 = feedback #1(TRUE) -> (w212:bool)
        n58 = Or(x=w213, y=w212) -> (x .or. y?=w211:bool)
        n59 = Select(t=w211, s="gen.burst/cont", f=w213) -> (s? t:f=w214:bool)
        n60 = call <instrlib>:"Synchronous Latch.vi"("clear"=w214, "set"=w210) -> ("out"=w215:bool)  [unwired: 9 in]
        n61 = And(x=w215, y="gen.triggered read") -> (x .and. y?=w229:bool)
        n62 = Or(x=w229, y="gen.read") -> (x .or. y?=w226:bool)
        n63 = call <instrlib>:"Detect Rising Edge.vi"("signal"=w226) -> ("edge detected"=w222:bool)  [unwired: 14 in]
        n64 = Or(x=w222, y=w212) -> (x .or. y?=w225:bool)
        n65 = call-poly <instrlib>:"Count Up.vi"("increment"=w215, "reset"=w225) -> ("count out"=w224:u16)  [unwired: 13 in]
        n66 = call-poly <instrlib>:"Count Up.vi"("increment"=w232, "reset"="gen.load") -> ("count out"=w235:u16)  [unwired: 13 in]
        n67 = Equal?(x=w224, y="gen.length") -> (x = y?=w238:bool)
        n68 = feedback-in #1(w238) -> ()
        n69 = feedback #2(FALSE ("gen mem.read")) -> (w241:bool)
        n70 = feedback-in #2(w226) -> ()
        n71 = feedback #3() -> (w242:u16)  [unwired: 1 in]
        n72 = feedback-in #3(w224) -> ()
        n73 = feedback #4(u16 0 ("count out")) -> (w234:u16)
        n74 = feedback-in #4(w235) -> ()
        n75 = call-poly <instrlib>:"Number Array To Boolean Array.vi"("data in"=w227) -> ("data out"=w243:bool[])  [unwired: 14 in]
        n76 = case shown="True" w241 {
          tunnel: w242 -> [_ w244]
          tunnel: [_ w245] -> w239
          frame False {
          }
          frame True {
            n77 = xnode ("Memory Method Node")("Address"=w244) -> ("Data"=w246:bool[])  [unwired: 1 in, 1 out]
            n78 = feedback #5() -> (w245:bool[])  [unwired: 1 in]
            n79 = feedback-in #5(w246) -> ()
          }
        }
        n80 = case shown="True" w232 {
          tunnel: w243 -> [_ w257]
          tunnel: w234 -> [_ w256]
          frame False {
          }
          frame True {
            n81 = xnode ("Memory Method Node")("Address"=w256, "Data"=w257) -> ()  [unwired: 1 in, 1 out]
          }
        }
        n82 = call-poly <instrlib>:"Boolean Array To Number Array.vi"("data in"=w239) -> ("data out"=w221:u32[])  [unwired: 14 in]
        n83 = Reshape Array(w221, 16 ("dimension size")) -> (w219:u32[])
        n84 = Split Number(x=w219) -> (hi(x)=w218:u16[], lo(x)=w217:u16[])
        n85 = for {
          tunnel: [w253] -> w209 mode=indexing
          tunnel: w218 -> [w252] mode=indexing
          tunnel: w217 -> [w251] mode=indexing
          w248 = fxp<+/-,16,1> 0.0 ("fixed-point type")
          n86 = Integer to Fixed-Point Cast(fixed-point type=w248, integer=w251) -> (fixed-point=w250:fxp<+/-,16,1>)
          n87 = Integer to Fixed-Point Cast(fixed-point type=w248, integer=w252) -> (fixed-point=w249:fxp<+/-,16,1>)
          n88 = To Fixed-Point(number=w249) -> (fixed-point=w255:fxp<+/-,18,1>)  [unwired: 1 in]
          n89 = To Fixed-Point(number=w250) -> (fixed-point=w254:fxp<+/-,18,1>)  [unwired: 1 in]
          n90 = Bundle By Name(cluster=T35 {"I"=0.0, "Q"=0.0, "overflow"=FALSE} ("data"), "I"=w255, "Q"=w254) -> (w253:T35)
        }
      }
      frame Enabled {
        # "generation becomes active on start trigger\nand gets inactive once there is no more\ndata available from memory"
        n91 = feedback-in #6(w274) -> ()
        n92 = feedback #6() -> (w264:bool)  [unwired: 1 in]
        n93 = And(x=w264, y="gen.enable") -> (x .and. y?=w262:bool)
        n94 = call <instrlib>:"Detect Rising Edge.vi"("signal"=w262) -> ("edge detected"=w273:bool)  [unwired: 14 in]
        n95 = local read "memo.reset"() -> (w272:bool)
        n96 = local read "flush"() -> (w268:bool)
        n97 = Or(x=w273, y=w272) -> (x .or. y?=w271:bool)
        n98 = local read "burst memo"() -> (w265:T2)
        n99 = Not(x=w268) -> (.not. x?=w267:bool)
        n100 = feedback #7() -> (w278:bool)  [unwired: 1 in]
        n101 = feedback #8() -> (w263:bool)  [unwired: 1 in]
        n102 = call <instrlib>:"Synchronous Latch.vi"("clear"=w263, "set"=w273) -> ("out"=w276:bool)  [unwired: 9 in]
        n103 = Compound Arithmetic op=AND(w276, w278) -> (w277:bool)
        n104 = Or(x=w268, y=w277) -> (x .or. y?=w269:bool)
        n105 = case shown="\"DRAM\", Default" w265 {
          tunnel: [w299 TRUE ("ready for input")] -> w279
          tunnel: [w293 w320] -> w260
          tunnel: w271 -> [w289 _]
          tunnel: [w288 w318] -> w270
          tunnel: w269 -> [w286 w316]
          tunnel: w267 -> [w285 w315]
          tunnel: w266 -> [w283 w314]
          tunnel: [w281 w311] -> w258
          frame "DRAM", Default {
            # "Retrieve next 512b content from memory\nout queue"
            # "512b to 384b\n- 16 IQ (12b)\nunpacking"
            n106 = Unbundle By Name(w283) -> ("DRAM read data FIFO"=w282:refnum<k21>)
            n107 = xnode ("FIFO Read Using Handshaking")("FIFO In"=w282) -> ("Number of Elements to Read"=w293:u32, "FIFO Out"=w280:refnum<k21>)
            n108 = xnode ("FIFO Read Using Handshaking")("Ready for Output"=w286, "FIFO In"=w280) -> ("Element"=w300:bool[], "Output Valid"=w287:bool)  [unwired: 1 out]
            n109 = And(x=w287, y=w285) -> (x .and. y?=w284:bool)
            n110 = call "512bit to 16 IQ samples unpack.vi"("reset"=w289, "input valid"=w284, "data in"=w300) -> ("output valid"=w281:bool, "data out"=w292:fxp<+/-,12,1>[], "ready for input"=w299:bool)  [unwired: 6 in]
            n111 = Select(t=w292, s=w281, f=fxp<+/-,12,1>[] [0.0, 0.0, 0.0, 0.0, 0.0, 0.0, 0.0, 0.0, 0.0, 0.0, 0.0, 0.0, 0.0, 0.0, 0.0, 0.0, 0.0, 0.0, 0.0, 0.0, 0.0, 0.0, 0.0, 0.0, 0.0, 0.0, 0.0, 0.0, 0.0, 0.0, 0.0, 0.0] ("data out")) -> (s? t:f=w291:fxp<+/-,12,1>[])
            n112 = feedback #9() -> (w298:fxp<+/-,12,1>[])  [unwired: 1 in]
            n113 = feedback-in #9(w291) -> ()
            n114 = Split 1D Array(array=w298, index=16) -> (first subarray=w296:fxp<+/-,12,1>[], second subarray=w295:fxp<+/-,12,1>[])
            n115 = for {
              N: 16 -> [_]
              tunnel: w296 -> [w303] mode=indexing
              tunnel: w295 -> [w302] mode=indexing
              tunnel: [w301] -> w288 mode=indexing
              # "2 x 12bit to\n DSP IQ (2 x 18bit)"
              n116 = To Fixed-Point(number=w303) -> (fixed-point=w306:fxp<+/-,18,1>)  [unwired: 1 in]
              n117 = To Fixed-Point(number=w302) -> (fixed-point=w305:fxp<+/-,18,1>)  [unwired: 1 in]
              n118 = Bundle By Name(cluster=T35 {"I"=0.0, "Q"=0.0, "overflow"=FALSE} ("data"), "I"=w306, "Q"=w305) -> (w301:T35)
            }
          }
          frame "BRAM" {
            # "#fpgatodo\ndocument and draw icon"
            # "448b to 16IQ (14bit)"
            # "Retrieve next 512b content from memory\nout queue"
            n119 = Unbundle By Name(w314) -> ("BRAM read data FIFO"=w313:refnum<k21>)
            n120 = xnode ("FIFO Read Using Handshaking")("FIFO In"=w313) -> ("Number of Elements to Read"=w320:u32, "FIFO Out"=w307:refnum<k21>)
            n121 = xnode ("FIFO Read Using Handshaking")("Ready for Output"=w316, "FIFO In"=w307) -> ("Element"=w310:bool[], "Output Valid"=w317:bool)  [unwired: 1 out]
            n122 = And(x=w317, y=w315) -> (x .and. y?=w311:bool)
            n123 = call "512bit to 16 IQ samples unpack (14bit).vi"("Element"=w310) -> ("Array"=w308:fxp<+/-,14,1>[])  [unwired: 10 in]
            n124 = Select(t=w308, s=w311, f=fxp<+/-,14,1>[] [0.0, 0.0, 0.0, 0.0, 0.0, 0.0, 0.0, 0.0, 0.0, 0.0, 0.0, 0.0, 0.0, 0.0, 0.0, 0.0, 0.0, 0.0, 0.0, 0.0, 0.0, 0.0, 0.0, 0.0, 0.0, 0.0, 0.0, 0.0, 0.0, 0.0, 0.0, 0.0] ("data out")) -> (s? t:f=w319:fxp<+/-,14,1>[])
            n125 = feedback #10() -> (w325:fxp<+/-,14,1>[])  [unwired: 1 in]
            n126 = feedback-in #10(w319) -> ()
            n127 = Split 1D Array(array=w325, index=16) -> (first subarray=w323:fxp<+/-,14,1>[], second subarray=w322:fxp<+/-,14,1>[])
            n128 = for {
              N: 16 -> [_]
              tunnel: w323 -> [w328] mode=indexing
              tunnel: w322 -> [w327] mode=indexing
              tunnel: [w326] -> w318 mode=indexing
              # "2 x 14bit to\n DSP IQ (2 x 18bit)"
              n129 = To Fixed-Point(number=w328) -> (fixed-point=w331:fxp<+/-,18,1>)  [unwired: 1 in]
              n130 = To Fixed-Point(number=w327) -> (fixed-point=w330:fxp<+/-,18,1>)  [unwired: 1 in]
              n131 = Bundle By Name(cluster=T35 {"I"=0.0, "Q"=0.0, "overflow"=FALSE} ("data"), "I"=w331, "Q"=w330) -> (w326:T35)
            }
          }
        }
        "gen.pending to read" <- w260
        n132 = feedback-in #7(w279) -> ()
        n133 = call-poly <instrlib>:"Count Up.vi"("increment"=w258, "reset"=w273) -> ("count out"=→"gen.total samples":u64)  [unwired: 13 in]
        n134 = Equal To 0?(x=w260) -> (x = 0?=w259:bool)
        n135 = feedback-in #8(w259) -> ()
      }
    }
    n136 = And(x=w107, y="gain ranging.enable") -> (x .and. y?=w185:bool)
    n137 = call "Aurora Send TX trigger data.vi"("start trigger"=w107, "aurora.write"="aurora.write", "aurora.reset trigger"="aurora.reset trigger", "clear overflow"="aurora.fifo overflow clear", "aurora tx fifo"=refnum<k21> "aurora tx fifo 0" ("FIFO In")) -> ("tx overflow latch"=→"aurora.fifo 0 overflow":bool, "trig count"=→"aurora.tx val":u16)  [unwired: 9 in]
    n138 = call "gain ranging test FSM.vi"("gain ranging.start sequence"=w185, "gain ranging.dwell time (cycles)"="gain ranging.dwell time (cycles)", "gain ranging.gain setting list"="gain ranging.setting list step", "gain ranging.manual request"="gain ranging.manual setting") -> ("gain ranging.gain setting"=w172:fxp<+/-,16,12>, "gain ranging.TX1/RX1 Port Value"=w169:T12, "gain ranging.gain setting valid"=w170:bool)  [unwired: 8 in, 1 out]
    n139 = call "Gain to Coarse Gain Index.vi"("gain setting"=w172, "coarse gain values"="gain ranging.coarse gain values") -> ("coarse gain index"=w176:u32)  [unwired: 13 in]
    n140 = call "Start trigger export.vi"("trig.pxi trig dst"="trig.pxi dst", "trig.export"="trig.export", "trig.dur"=u32 25, "delayed trigger"=w117, "synced trigger"=w107, "source trigger"=w118) -> ()  [unwired: 2 in, 4 out]
    n141 = feedback #11() -> (w174:fxp<+/-,16,12>)  [unwired: 1 in]
    n142 = feedback-in #11(w172) -> ()
    n143 = feedback #12() -> (w157:bool)  [unwired: 1 in]
    n144 = feedback-in #12(w170) -> ()
    n145 = feedback #13() -> (w166:u32)  [unwired: 1 in]
    n146 = feedback-in #13(w176) -> ()
    n147 = feedback #14() -> (w168:T12)  [unwired: 1 in]
    n148 = feedback-in #14(w169) -> ()
    n149 = And(x="gain ranging.enable fine gain ranging", y=w157) -> (x .and. y?=w173:bool)
    n150 = And(x="gain ranging.enable coarse gain ranging", y=w157) -> (x .and. y?=w165:bool)
    n151 = And(x="gain ranging.enable port config", y=w157) -> (x .and. y?=w158:bool)
    n152 = feedback #15() -> (w141:bool)  [unwired: 1 in]
    n153 = call "20 kHz TClk Counter.vi"("master 10 kHz reset"=w141, "tclk"=w153, "20 kHz tclk parameters"="20 kHz tclk parameters") -> ("tclk offset value"=→"tclk value":u16)  [unwired: 12 in]
    n154 = call "Sysref offset counter.vi"("master 10 kHz reset"=w141) -> ("sysref offset value"=→"sysref value":u8)  [unwired: 14 in]
    n155 = disable-structure shown="Enabled" {
      disable-tunnel: w158 -> [w352 w361]
      disable-tunnel: w168 -> [w351 w360]
      disable-tunnel: "gain ranging.enable port config" -> [w348 w356]
      disable-tunnel: w154 -> [w347 w355]
      frame Enabled {
        w350 = refnum<k21> "PXIe_DStarC" ("FPGA I/O In")
        # "Do not remove\nHandles trigger hold-off"
        # "Configure mmWave Port - re-use trig 6"
        # "Pass-through resource"
        # "Arbitration is only required when using Trig 6, other triggers can be accessed normally. Trig 4 is reserved for runtime synchronization"
        n156 = call <instrlib>:"Configure mmWave Port.vi"("port"=w351, "pxi trigger"=w350, "input valid"=w352) -> ()  [unwired: 12 in, 1 out]
        n157 = xnode "FPGA I/O Node"("FPGA I/O In"=w350) -> ("I/O Item"=w349:bool)  [unwired: 1 out]
        n158 = Bundle By Name(cluster=T36 {"disable TClk measure"=FALSE, "output enable"=FALSE, "output value"=FALSE} ("pxi trig 6 arbiter"), "output enable"=w348, "output value"=w349, "disable TClk measure"=w347) -> (w353:T36)
        n159 = global write "Globals.vi" "pxi trig 6 arbiter"(w353) -> ()
      }
      frame Disabled {
        w359 = FALSE ("disable TClk measure")
        # "Note: this configuration is preferred but \nuses an additional trigger line"
        # "Config mmWave Port - dedicated trigger"
        # "Arbitration is only required when using Trig 6, other triggers can be accessed normally. Trig 4 is reserved for runtime synchronization"
        n160 = xnode "FPGA I/O Method Node"("FPGA I/O In"=refnum<k21> "PXI_Trig0" ("pxi trigger 1"), "Enable"=w356) -> ("FPGA I/O Out"=w358:refnum<k21>)
        n161 = call <instrlib>:"Configure mmWave Port.vi"("port"=w360, "pxi trigger"=w358, "input valid"=w361) -> ()  [unwired: 12 in, 1 out]
        n162 = Bundle By Name(cluster=T36 {"disable TClk measure"=FALSE, "output enable"=FALSE, "output value"=FALSE} ("pxi trig 6 arbiter"), "output value"=w359, "output enable"=w359, "disable TClk measure"=w355) -> (w362:T36)
        n163 = global write "Globals.vi" "pxi trig 6 arbiter"(w362) -> ()
      }
    }
    n164 = global read "Globals.vi" "txjesd.control"() -> (w162:T15)
    n165 = global read "Globals.vi" "txjesd.control"() -> (w189:T15)
    n166 = Unbundle By Name(w162) -> ("trig7 listen"=w145:bool)
    n167 = disable-structure shown="Enabled" {
      disable-tunnel: "tone.routing" -> [w198 _]
      disable-tunnel: "tone.parameters" -> [w197 _]
      disable-tunnel: [w195 _] -> w108
      disable-tunnel: w107 -> [w194 _]
      frame Disabled {
        n168 = call "Multi-tone Generator.vi"("tone.parameters"=w197, "tone.reset"=w194, "tone routing"=w198, "input valid"=TRUE) -> ("tone data"=w195:T35[])  [unwired: 10 in, 1 out]
      }
      frame Enabled {
      }
    }
    n169 = Unbundle By Name(w189) -> ("clear data in error"=w190:bool)
    n170 = Compound Arithmetic op=AND(invert w145, invert "sync.master reset listen", "gain ranging.enable coarse gain ranging") -> (w161:bool)
    n171 = xnode "FPGA I/O Method Node"("FPGA I/O In"=refnum<k21> "PXI_Trig5" ("pxi trigger 1"), "Enable"="gain ranging.enable coarse gain ranging") -> ("FPGA I/O Out"=w164:refnum<k21>)
    n172 = xnode "FPGA I/O Method Node"("FPGA I/O In"=refnum<k21> "PXI_Trig7" ("pxi trigger 1"), "Enable"=w161) -> ("FPGA I/O Out"=w163:refnum<k21>)
    n173 = Or(x=w145, y="sync.master reset listen") -> (x .or. y?=w148:bool)
    n174 = case shown="\"Waveform Generation\"" "waveform type" {
      tunnel: w108 -> [w199 _]
      tunnel: [w199 w200] -> w112
      tunnel: w106 -> [_ w200]
      frame "Tone", Default {
      }
      frame "Waveform Generation" {
      }
    }
    n175 = case shown="True" FALSE {
      tunnel: [FALSE ("Timed Out?") w366] -> w181
      tunnel: refnum<k21> "aurora tx fifo 1" ("FIFO In") -> [_ w365]
      frame False {
      }
      frame True {
        n176 = disable-structure shown="Disabled" {
          disable-tunnel: [w370 _] -> w366
          disable-tunnel: _ -> [w369 _]
          disable-tunnel: w365 -> [w367 _]
          frame Disabled {
            n177 = xnode ("FIFO Method Node")("Element"=w369, "Timeout"=0, "FIFO In"=w367) -> ("Timed Out?"=w370:bool)  [unwired: 1 out]
          }
          frame Enabled {
          }
        }
      }
    }
    n178 = call <instrlib>:"Write gain setting (Fine).vi"("gain"=w174, "table info"="table info", "P2P Writer FIFO"=refnum<k21> "P2P FIFO to PXIe-3620" ("FIFO In"), "direction"=enum8{"rx", "tx"}."tx", "input valid"=w173) -> ()  [unwired: 10 in, 1 out]
    n179 = disable-structure shown="Enabled" {
      disable-tunnel: "filter.coefficients" -> [w205 _]
      disable-tunnel: w112 -> [w203 w208]
      disable-tunnel: [w202 w208] -> w113
      disable-tunnel: "filter.enable" -> [w201 _]
      frame Enabled {
        n180 = call "EQ Parallel - 16 spc - 2x oc - 32 coef.vi"("data in"=w203, "clock x2"=refnum<k21> "7902R IO Socket\\SampleClkx2", "filter coefficients"=w205, "input valid"=TRUE) -> ("data out"=w204:T35[])  [unwired: 9 in, 2 out]
        n181 = Select(t=w204, s=w201, f=w203) -> (s? t:f=w202:T35[])
      }
      frame Disabled {
        # "optional equalizer disabled"
      }
    }
    n182 = case shown="True" w148 {
      tunnel: w163 -> [w336 w339]
      tunnel: w164 -> [w335 _]
      tunnel: w166 -> [w334 _]
      tunnel: w165 -> [w333 _]
      tunnel: w162 -> [_ w340]
      tunnel: "sync.master reset listen" -> [_ w338]
      tunnel: [FALSE ("Master10k_Reset") w337] -> w144
      frame False {
        # "Coarse Gain Ranging - not required"
        n183 = call <instrlib>:"Write gain setting (Coarse).vi"("fast jump table index"=w334, "pxi trigger 1"=w335, "pxi trigger 2"=w336, "input valid"=w333) -> ()  [unwired: 11 in, 1 out]
      }
      frame True {
        # "Depending on the active signal\ndo JESD sync or receive\nmaster 10 kHz reset"
        # "JESD Sync - required"
        n184 = xnode "FPGA I/O Node"("FPGA I/O In"=w339) -> ("I/O Item"=w341:bool)  [unwired: 1 out]
        n185 = case shown="True" w338 {
          tunnel: w341 -> [w344 w346]
          tunnel: w340 -> [w343 _]
          tunnel: [FALSE ("Master10k_Reset") w345] -> w337
          frame False {
            n186 = call "TX JESD.vi"("txjesd.control"=w343, "trigger value"=w344) -> ()  [unwired: 14 in]
          }
          frame True {
            n187 = call "Master 10 kHz Reset.vi"("I/O Item"=w346) -> ("master 10 kHz reset"=w345:bool)  [unwired: 10 in]
          }
        }
      }
    }
    n188 = And(x="sync.counter reset enable", y=w144) -> (x .and. y?=w143:bool)
    n189 = feedback-in #15(w143) -> ()
    n190 = call <instrlib>:"Synchronous Latch.vi"("set"=w181) -> ("out"=→"aurora.fifo 1 overflow":bool)  [unwired: 10 in]
    n191 = call "Output Data.vi"("input data"=w113, "reset"=w107, "cal parameters"="cal.correction", "generation parameters"="cal.generation", "txjesd.clear data in error"=w190) -> ("txjesd.data in error"=w188:bool)  [unwired: 10 in]
    n192 = global write "Globals.vi" "data error"(w188) -> ()
  }
  n193 = node-c288() -> (w35:T29)  [unwired: 1 in]
  n194 = node-c288() -> (w56:T29)  [unwired: 1 in]
  n195 = timed-loop {
    timing: w35 -> [_]
    timing-out: [_] -> w34
    tunnel: w32 -> [w387]
    tunnel: w33 -> [w386]
    stop <- _ stop-if-true
    # "Single Port - 5.5GB/s"
    n196 = call "Aurora Reader (Single Port) .vi"("AXI4-Stream Reader FXP64x4"=w386) -> ("data"=w384:bool[], "output valid"=w383:bool)  [unwired: 13 in]
    n197 = case shown="True" w383 {
      tunnel: w384 -> [_ w395]
      tunnel: [FALSE ("Timed Out?") w393] -> w382
      frame False {
      }
      frame True {
        n198 = xnode ("FIFO Write")("Element"=w395, "Timeout"=0) -> ("Timed Out?"=w393:bool)  [unwired: 1 in, 1 out]
      }
    }
    n199 = call <instrlib>:"Synchronous Latch.vi"("clear"="port 4.rx fifo overflow clear", "set"=w382) -> ("out"=→"port 4.rx fifo overflow":bool)  [unwired: 9 in]
    n200 = call "Aurora Read Debug Signals (Single Port).vi"("Debug CLIP Resources"=T37 {"Hard Error"="7902R IO Socket\\uPort4_HardError", "Soft Error"="7902R IO Socket\\uPort4_SoftError", "Lane Up"="7902R IO Socket\\uPort4_LaneUp", "Channel Up"="7902R IO Socket\\uPort4_ChannelUp", "Sys Reset"="7902R IO Socket\\uPort4_sys_reset_out"}) -> ("Debug Info"=→"port 4.debug info":T9)  [unwired: 14 in]
    n201 = feedback #16(FALSE ("ready for input")) -> (w376:bool)
    n202 = case shown="True" w376 {
      tunnel: [_ w391] -> w385
      tunnel: [TRUE ("Timed Out?") w390] -> w379
      frame False {
      }
      frame True {
        n203 = xnode ("FIFO Method Node")("Timeout"=0) -> ("Element"=w391:bool[], "Timed Out?"=w390:bool)  [unwired: 1 in, 1 out]
      }
    }
    n204 = Not(x=w379) -> (.not. x?=w378:bool)
    n205 = call "Aurora Writer (Single Port).vi"("input data"=w385, "AXI4-Stream Writer FXP64x4"=w387, "input valid"=w378) -> ("ready for input"=w377:bool)  [unwired: 12 in]
    n206 = feedback-in #16(w377) -> ()
  }
  n207 = timed-loop {
    timing: w56 -> [_]
    timing-out: [_] -> w55
    stop <- _ stop-if-true
    # "CLIP Control and Status"
    n208 = Unbundle By Name("txjesd.control") -> ("reset"=w409:bool, "gtx enable"=w408:bool, "jesd enable"=w407:bool, "sw sync"=w406:bool, "gtx post cursor"=w405:fxp<+,5,5>, "gtx pre cursor"=w404:fxp<+,5,5>, "gtx diff control"=w403:fxp<+,4,4>, "clock enable"=w402:bool, "lmfc delay"=w401:fxp<+,5,5>)
    n209 = global write "Globals.vi" "txjesd.control"("txjesd.control") -> ()
    n210 = xnode "FPGA I/O Node"("7902R IO Socket\\aResetSl"=w409, "7902R IO Socket\\aGtxEnable"=w408, "7902R IO Socket\\aJesdEnable"=w407, "7902R IO Socket\\aSyncFromSw"=w406, "7902R IO Socket\\aGtxPostCursor"=w405, "7902R IO Socket\\aGtxPreCursor"=w404, "7902R IO Socket\\aGtxDiffCntrl"=w403, "7902R IO Socket\\aClkEnable"=w402, "7902R IO Socket\\aLmfcDly"=w401) -> ()  [unwired: 9 in, 9 out]
    n211 = xnode "FPGA I/O Node"() -> ("7902R IO Socket\\aGtxActive"=w419:bool, "7902R IO Socket\\aJesdActive"=w413:bool, "7902R IO Socket\\aLaneSyncReq"=w414:bool, "7902R IO Socket\\aLanesSynced"=w415:bool, "7902R IO Socket\\aLanesAligned"=w416:bool, "7902R IO Socket\\aQpllLocked"=w417:bool, "7902R IO Socket\\aQpllRefLost"=w418:bool, "7902R IO Socket\\MgtRefClks_Locked"=w411:bool, "7902R IO Socket\\MgtRefClks_Valid"=w410:bool)  [unwired: 9 in, 9 out]
    n212 = global read "Globals.vi" "data error"() -> (w398:bool)
    n213 = Bundle By Name(cluster=T16 {"gtx active"=FALSE, "jesd active"=FALSE, "lane sync req"=FALSE, "lanes synced"=FALSE, "lanes aligned"=FALSE, "qpll locked"=FALSE, "qpll ref lost"=FALSE, "mgt ref clocks locked"=FALSE, "mgt ref clock valid"=FALSE, "data error"=FALSE} ("txjesd.status 2"), "gtx active"=w419, "jesd active"=w413, "lane sync req"=w414, "lanes synced"=w415, "lanes aligned"=w416, "qpll locked"=w417, "qpll ref lost"=w418, "mgt ref clocks locked"=w411, "mgt ref clock valid"=w410, "data error"=w398) -> (→"txjesd.status":T16)
  }
  n214 = node-c288(w34) -> ()
  n215 = disable-structure shown="Disabled" {
    frame Disabled {
      n216 = node-c288 ("Input Node")() -> (w427:T29)  [unwired: 1 in]
      n217 = call "Aurora Create Resources (Single Port).vi"("RX CLIP Resources"=T28 {"m_axis_tvalid"="7902R IO Socket\\uPort5_m_axi_rx_tvalid", "m_axis_tdata_0"="7902R IO Socket\\uPort5_m_axi_rx_tdata_0", "m_axis_tdata_1"="7902R IO Socket\\uPort5_m_axi_rx_tdata_1", "m_axis_tdata_2"="7902R IO Socket\\uPort5_m_axi_rx_tdata_2", "m_axis_tdata_3"="7902R IO Socket\\uPort5_m_axi_rx_tdata_3"}, "TX CLIP Resources"=T27 {"s_axis_tvalid"="7902R IO Socket\\uPort5_s_axi_tx_tvalid", "s_axis_tdata_0"="7902R IO Socket\\uPort5_s_axi_tx_tdata_0", "s_axis_tdata_1"="7902R IO Socket\\uPort5_s_axi_tx_tdata_1", "s_axis_tdata_2"="7902R IO Socket\\uPort5_s_axi_tx_tdata_2", "s_axis_tdata_3"="7902R IO Socket\\uPort5_s_axi_tx_tdata_3", "s_axis_tready"="7902R IO Socket\\uPort5_s_axi_tx_tready"}) -> ("AXI4-Stream Reader FXP64x4"=w425:T33, "AXI4-Stream Writer FXP64x4"=w424:T34)  [unwired: 8 in]
      n218 = timed-loop {
        timing: w427 -> [_]
        timing-out: [_] -> w426
        tunnel: w424 -> [w428]
        tunnel: w425 -> [w432]
        stop <- _ stop-if-true
        # "Single Port - 5.5GB/s"
        n219 = call "Aurora Reader (Single Port) .vi"("AXI4-Stream Reader FXP64x4"=w432) -> ("data"=w434:bool[], "output valid"=w433:bool)  [unwired: 13 in]
        n220 = case shown="True" w433 {
          tunnel: w434 -> [_ w450]
          tunnel: [FALSE ("Timed Out?") w449] -> w440
          frame False {
          }
          frame True {
            n221 = xnode ("FIFO Method Node")("Element"=w450, "Timeout"=0) -> ("Timed Out?"=w449:bool)  [unwired: 1 in, 1 out]
          }
        }
        n222 = call <instrlib>:"Synchronous Latch.vi"("clear"="port 5.rx fifo overflow clear", "set"=w440) -> ("out"=→"port 5.rx fifo overflow":bool)  [unwired: 9 in]
        n223 = call "Aurora Read Debug Signals (Single Port).vi"("Debug CLIP Resources"=T37 {"Hard Error"="7902R IO Socket\\uPort5_HardError", "Soft Error"="7902R IO Socket\\uPort5_SoftError", "Lane Up"="7902R IO Socket\\uPort5_LaneUp", "Channel Up"="7902R IO Socket\\uPort5_ChannelUp", "Sys Reset"="7902R IO Socket\\uPort5_sys_reset_out"}) -> ("Debug Info"=→"port 5.debug info":T9)  [unwired: 14 in]
        n224 = feedback #17(FALSE ("ready for input")) -> (w436:bool)
        n225 = case shown="True" w436 {
          tunnel: [_ w446] -> w431
          tunnel: [TRUE ("Timed Out?") w445] -> w437
          frame False {
          }
          frame True {
            n226 = xnode ("FIFO Method Node")("Timeout"=0) -> ("Element"=w446:bool[], "Timed Out?"=w445:bool)  [unwired: 1 in, 1 out]
          }
        }
        n227 = Not(x=w437) -> (.not. x?=w430:bool)
        n228 = call "Aurora Writer (Single Port).vi"("input data"=w431, "AXI4-Stream Writer FXP64x4"=w428, "input valid"=w430) -> ("ready for input"=w429:bool)  [unwired: 12 in]
        n229 = feedback-in #17(w429) -> ()
      }
      n230 = node-c288(w426) -> ()
    }
    frame Enabled {
    }
  }
  n231 = node-c288(w55) -> ()
  n232 = xnode "VI-Defined Handshake"() -> ("Handshake Out"=w48:refnum<k21>)
  n233 = xnode "VI-Defined Handshake"() -> ("Handshake Out"=w47:refnum<k21>)
  n234 = xnode "VI-Defined Handshake"() -> ("Handshake Out"=w45:refnum<k21>)
  n235 = xnode "VI-Defined Handshake"() -> ("Handshake Out"=w41:refnum<k21>)
  n236 = xnode "VI-Defined Handshake"() -> ("Handshake Out"=w42:refnum<k21>)
  n237 = xnode "VI-Defined Handshake"() -> ("Handshake Out"=w39:refnum<k21>)
  n238 = xnode "VI-Defined Handshake"() -> ("Handshake Out"=w38:refnum<k21>)
  n239 = node-c288() -> (w51:T29)  [unwired: 1 in]
  n240 = call "Monitor Clock Process.vi"("clock name"=refnum<k21> "40 MHz Onboard Clock", "handshake"=w48) -> ()  [unwired: 14 in]
  n241 = call "Monitor Clock Process.vi"("clock name"=refnum<k21> "100 MHz Clock", "handshake"=w47) -> ()  [unwired: 14 in]
  n242 = call "Monitor Clock Process.vi"("clock name"=refnum<k21> "7902R IO Socket\\SampleClk", "handshake"=w45) -> ()  [unwired: 14 in]
  n243 = call "Monitor Clock Process.vi"("clock name"=refnum<k21> "7902R IO Socket\\SampleClkx2", "handshake"=w41) -> ()  [unwired: 14 in]
  n244 = call "Monitor Clock Process.vi"("clock name"=refnum<k21> "7902R IO Socket\\SampleClkDiv2", "handshake"=w42) -> ()  [unwired: 14 in]
  n245 = call "Monitor Clock Process.vi"("clock name"=refnum<k21> "7902R IO Socket\\Port4_UserClk", "handshake"=w39) -> ()  [unwired: 14 in]
  n246 = call "Monitor Clock Process.vi"("clock name"=refnum<k21> "7902R IO Socket\\Port5_UserClk", "handshake"=w38) -> ()  [unwired: 14 in]
  n247 = timed-loop {
    timing: w51 -> [_]
    timing-out: [_] -> w50
    tunnel: w48 -> [w469]
    tunnel: w47 -> [w468]
    tunnel: w45 -> [w464]
    tunnel: w41 -> [w461]
    tunnel: w42 -> [w462]
    tunnel: w39 -> [w458]
    tunnel: w38 -> [w457]
    stop <- _ stop-if-true
    n248 = call "Get Clock State.vi"("handshake in"=w469) -> ("clock valid"=w467:bool)  [unwired: 14 in]
    n249 = call "Get Clock State.vi"("handshake in"=w468) -> ("clock valid"=w466:bool)  [unwired: 14 in]
    n250 = call "Get Clock State.vi"("handshake in"=w464) -> ("clock valid"=w463:bool)  [unwired: 14 in]
    n251 = call "Get Clock State.vi"("handshake in"=w461) -> ("clock valid"=w460:bool)  [unwired: 14 in]
    n252 = call "Get Clock State.vi"("handshake in"=w462) -> ("clock valid"=w459:bool)  [unwired: 14 in]
    n253 = call "Get Clock State.vi"("handshake in"=w458) -> ("clock valid"=w456:bool)  [unwired: 14 in]
    n254 = call "Get Clock State.vi"("handshake in"=w457) -> ("clock valid"=w455:bool)  [unwired: 14 in]
    n255 = Build Array(w467, w466, w463, w460, w459, w456, w455) -> (→"clocks valid":bool[])
  }
  n256 = node-c288(w50) -> ()
  n257 = node-c288(w53) -> ()
